vi "Get GUID.vi"(11 "Messenger in":refnum<class "Messenger.lvclass">) -> (2 "GUID":string, 3 "Messenger out":refnum<class "Messenger.lvclass">)   [LabVIEW 2014, in "Messenger.lvclass"]
uses:
  Messenger.lvclass
  Messenger.lvclass/Messenger.ctl
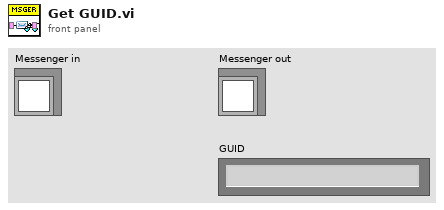
[diagram p1: front panel]
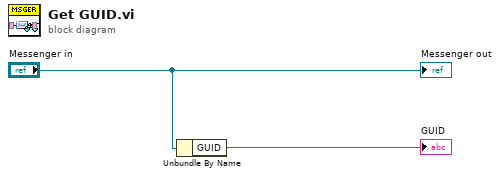
[diagram p0: block diagram]
diagram:
  n1 = Unbundle By Name("Messenger in") -> ("GUID"=→"GUID":string)
  "Messenger out" <- "Messenger in"
